vi "Activation.vi"() -> ()   [LabVIEW 2013, in "main.lvlib"]
uses:
  main.lvlib
  Controls/Enum Save Action Events.ctl
  Controls/Enum Variables.ctl
panel:
  in  "ActivateDicom_CancelBtn":bool
  out "ActivateDicom_TitleString":string="Aktiver DICOM"
  in  "ActivateBtn":bool
  out "Hospital:":string
  in  "Licens":string
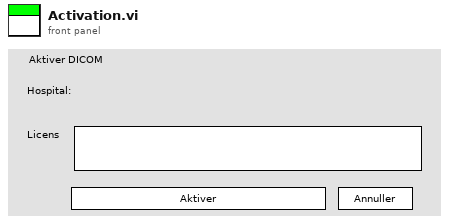
[diagram p1: front panel]
types:
  T1 = typedef "main.lvlib/Enum Variables.ctl" = enum16{"SetAcqFilter", "GetAcqFilter", "Set Filter", "Get Filter", "Set Height", "Get Height", "Set Recorded Height", "Get Recorded Height", "Set Blue Pressure", "Get Blue Pressure", "Set Red Pressure", "Get Red Pressure", "Init", "Reset Pressure", "Set Red Cursors", "Get Red Cursors", "Set Blue Cursors", "Get Blue Cursors", "Set Language", "Get Language", "Set Active Graphs", "Get ActiveGraphs", "Set Method", "Get Method", "Set Encryption", "Get Encryption", "Set ExcelVersion", "Get ExcelVersion", "Set DICOM Avail", "Get DICOM Avail", "Set DICOM Encode", "Get DICOM Encode", "Set JournalExport", "Get JournalExport", "Set Sequence", "Get Sequence", "Set DAQ Connected", "Get DAQ Connected", "Set Current Graph", "Get Current Graph", "Set General Settings", "Get Hyphenation", "Set Arm Calc Method", "Get Arm Calc Method", "Set Dicom Tags", "Get Dicom Tags", "Set BT Serial", "Get BT Serial", "Set BT Accepted Serials", "Get BT Accepted Serials", "Get BT License", "Set BT License"}
  T2 = cluster{"Name":string, "Address":string, "Department":string}
  T3 = typedef "main.lvlib/Enum Save Action Events.ctl" = enum16{"LoadReportPath", "SaveReportPath", "Load Graph Path", "Save Graph Path", "LoadDataPath", "SaveDataPath", "Load Template Path", "Save Template Path", "Load PressureFactor", "Save PressureFactor", "Init", "Load Listbox", "Save Listbox", "LoadHospInfo", "SaveHospInfo", "Load DICOM Activation", "Save DICOM Activation", "LoadDICOMInfoWL", "SaveDICOMInfoWL", "LoadDICOMInfoPACS", "SaveDICOMInfoPACS", "Load ArmCalcMethod", "Save ArmCalcMethod", "LoadItemTags", "SaveItemTags", "LoadDICOMEncoding", "SaveDICOMEncoding", "LoadJournalType", "SaveJournalType", "LoadAcqFilterType", "SaveAcqFilterType", "Load Sequence", "Save Sequence", "Load Acquisition Mode", "Save Acquisition Mode", "Load General Settings", "Save General Settings", "Load Language", "Save Language", "Load Dicom Tags", "Save Dicom Tags", "Load BT Serial", "Save BT Serial", "Load BT License", "Save BT License"}
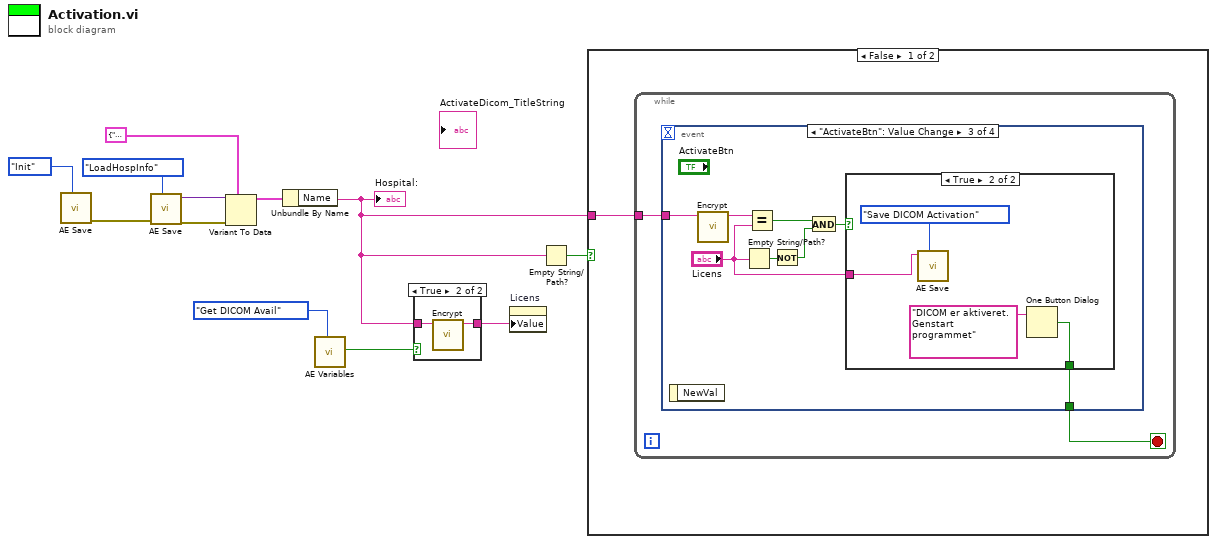
[diagram p0: block diagram]
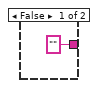
[diagram p2: hidden frame]
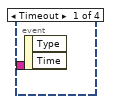
[diagram p3: hidden frame]
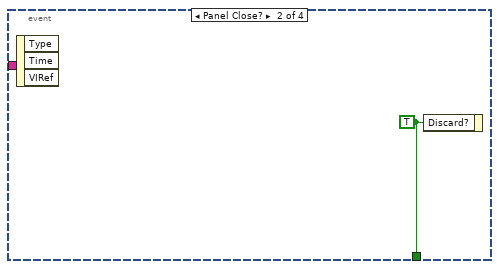
[diagram p4: hidden frame]
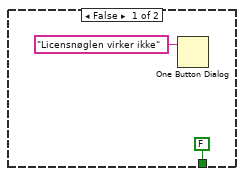
[diagram p5: hidden frame]
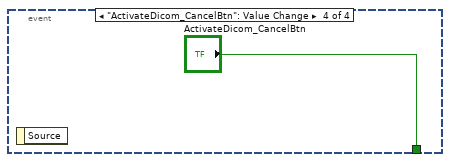
[diagram p6: hidden frame]
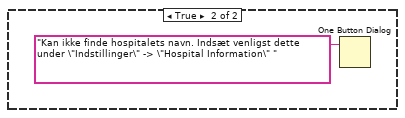
[diagram p7: hidden frame]
diagram:
  n1 = call "AE Save.vi"("Action"=Enum_Save_Action_Events."Init") -> ("error out"=w11:errorcluster)  [unwired: 8 in, 1 out]
  n2 = call "AE Save.vi"("error in (no error)"=w11, "Action"=Enum_Save_Action_Events."LoadHospInfo") -> ("error out"=w6:errorcluster, "Anything"=w7:variant)  [unwired: 7 in]
  n3 = Variant To Data(error in=w6, type=T2 {"Name"="", "Address"="", "Department"=""} ("HospInfo"), Variant=w7) -> (data=w8:T2)  [unwired: 1 out]
  n4 = Unbundle By Name(w8) -> ("Name"=w2:string)
  "Hospital:" <- w2
  n5 = call "AE Variables.vi"("Action"=Enum_Variables."Get DICOM Avail") -> ("BooleanOut"=w1:bool)  [unwired: 11 in, 7 out]
  n6 = case shown="True" w1 {
    tunnel: ["" ("Output") w15] -> w3
    tunnel: w2 -> [_ w14]
    frame False {
    }
    frame True {
      n7 = call "Encrypt.vi"("Input"=w14) -> ("Output"=w15:string)  [unwired: 10 in]
    }
  }
  n8 = property on="Licens" class="Str"("Value"=w3) -> ()  [unwired: 2 in, 2 out]
  n9 = Empty String/Path?(string/path=w2) -> (empty?=w5:bool)
  n10 = case shown="False" w5 {
    tunnel: w2 -> [w16 _]
    frame False {
      n11 = while {
        tunnel: w16 -> [w17]
        stop <- w18 stop-if-true
        n12 = event shown="[2] \"ActivateBtn\": Value Change" {
          selector: _ -> [_ _ _ _]
          dyn-events: _ -> [_ _ _ _]
          timeout: _ -> [_ _ _ _]
          tunnel: [_ w19 w21 "ActivateDicom_CancelBtn"] -> w18
          tunnel: w17 -> [_ _ w27 _]
          event Timeout {
            n13 = event-data() -> ()  [unwired: 1 in, 2 out]
          }
          event Panel Close? {
            w19 = TRUE ("Discard?")
            n14 = event-data() -> ()  [unwired: 1 in, 3 out]
            n15 = event-data("Discard?"=w19) -> ()  [unwired: 1 in, 1 out]
          }
          event "ActivateBtn": Value Change {
            n16 = event-data() -> ()  [unwired: 1 in, 1 out]
            n17 = call "Encrypt.vi"("Input"=w27) -> ("Output"=w26:string)  [unwired: 10 in]
            n18 = Empty String/Path?(string/path="Licens") -> (empty?=w25:bool)
            n19 = Equal?(x=w26, y="Licens") -> (x = y?=w23:bool)
            n20 = Not(x=w25) -> (.not. x?=w24:bool)
            n21 = And(x=w23, y=w24) -> (x .and. y?=w22:bool)
            n22 = case shown="True" w22 {
              tunnel: [FALSE w32] -> w21
              tunnel: "Licens" -> [_ w30]
              frame False {
                n23 = One Button Dialog(message="Licensnøglen virker ikke") -> ()  [unwired: 1 in, 1 out]
              }
              frame True {
                n24 = call "AE Save.vi"("Variant In"=w30, "Action"=Enum_Save_Action_Events."Save DICOM Activation") -> ()  [unwired: 7 in, 2 out]
                n25 = One Button Dialog(message="DICOM er aktiveret. Genstart programmet") -> (true=w32:bool)  [unwired: 1 in]
              }
            }
          }
          event "ActivateDicom_CancelBtn": Value Change {
            n26 = event-data() -> ()  [unwired: 1 in, 1 out]
          }
        }
      }
    }
    frame True {
      n27 = One Button Dialog(message="Kan ikke finde hospitalets navn. Indsæt venligst dette under \"Indstillinger\" -> \"Hospital Information\" ") -> ()  [unwired: 1 in, 1 out]
    }
  }
